vi "GetPivotSystemActual.vi"(9 "Relative Encoders?":bool, 10 "Zero Relative Encoder":bool, 11 "Zero Drive Encoder":bool) -> (3 "Robot Motion Commands Out":T1)   [LabVIEW 2018]
uses:
  Controls/Robot Pivot Motion Commands.ctl
  Controls/Pivot Motor Commands.ctl
  Controls/Robot Drive Mode.ctl
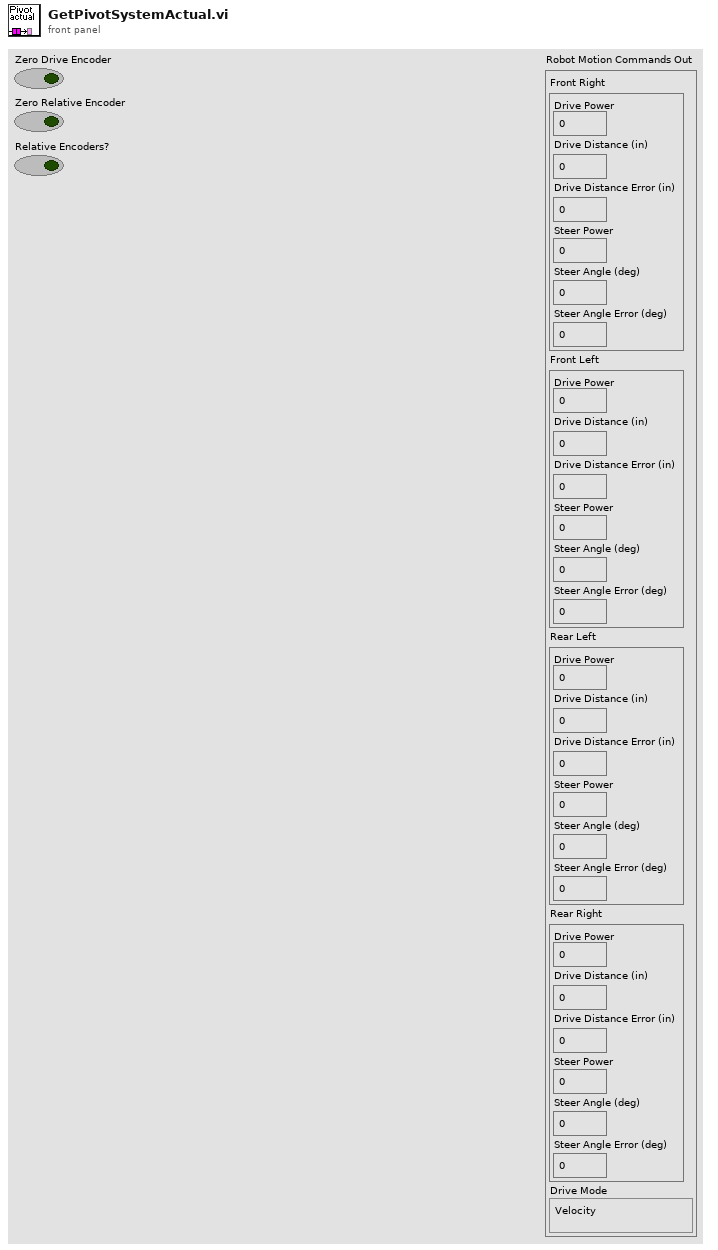
[diagram p1: front panel]
types:
  T1 = typedef "Robot Pivot Motion Commands.ctl" = cluster{"Front Right":T2, "Front Left":T2, "Rear Left":T2, "Rear Right":T2, "Drive Mode":T3}
  T2 = typedef "Pivot Motor Commands.ctl" = cluster{"Drive Power":dbl, "Drive Distance (in)":dbl, "Drive Distance Error (in)":dbl, "Steer Power":dbl, "Steer Angle (deg)":dbl, "Steer Angle Error (deg)":dbl}
  T3 = typedef "Robot Drive Mode.ctl" = enum16{"Velocity", "Distance"}
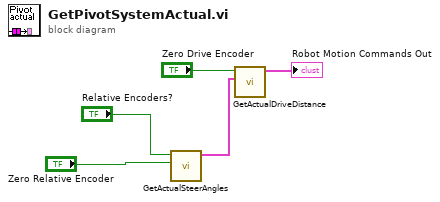
[diagram p0: block diagram]
diagram:
  n1 = call "GetActualSteerAngles.vi"("Zero Relative Encoder"="Zero Relative Encoder", "Relative Encoders?"="Relative Encoders?") -> ("Robot Motion Commands"=w5:T1)  [unwired: 9 in]
  n2 = call "GetActualDriveDistance.vi"("Robot Motion Commands In"=w5, "Zero Encoder"="Zero Drive Encoder") -> ("Robot Motion Commands Out"=→"Robot Motion Commands Out":T1)  [unwired: 7 in]
